vi "PathPlanner_Trajectory_GenerateStates_Pass3.vi"(9 "StartingSpeeds":T1 {"vOmega" format="%10.3f"; "vY" format="%10.3f"; "vX" format="%10.3f"}, 11 "in PathPlannerStates":T2[](array[typedef]) {"TargetHolonomicRotation"."SIN" format="%13.4f"; "TargetHolonomicRotation"."COS" format="%13.4f"; "TargetHolonomicRotation"."VALUE" format="%13.4f"; "Heading"."SIN" format="%13.4f"; "Heading"."COS" format="%13.4f"; "Heading"."VALUE" format="%13.4f"; "PositionMeters"."Y" format="%14.3f"; "PositionMeters"."X" format="%14.3f"}) -> (3 "out PathPlannerStates":T2[](array[typedef]) {"TargetHolonomicRotation"."SIN" format="%13.4f"; "TargetHolonomicRotation"."COS" format="%13.4f"; "TargetHolonomicRotation"."VALUE" format="%13.4f"; "Heading"."SIN" format="%13.4f"; "Heading"."COS" format="%13.4f"; "Heading"."VALUE" format="%13.4f"; "PositionMeters"."Y" format="%14.3f"; "PositionMeters"."X" format="%14.3f"})   [LabVIEW 2019, in "PathPlanner.lvlib"]
uses:
  PathPlanner.lvlib
  TypeDef/PathPlannerTrajectoryState.ctl
  <vilib>/Rock Robotics/WPI/ThirdParty/JAS_Junk/TrajLib/TypeDef/TRANSLATION2D.ctl
  <vilib>/Rock Robotics/WPI/ThirdParty/JAS_Junk/TrajLib/TypeDef/ROTATION2D.ctl
  TypeDef/PathPlannerPathConstraints.ctl
  <vilib>/Rock Robotics/WPI/ThirdParty/JAS_Junk/TrajLib/TypeDef/CHASSIS_SPEEDS.ctl
  <vilib>/Rock Robotics/WPI/ThirdParty/JAS_Junk/TrajLib/Rotation2d_UnaryMinus.vi
  <vilib>/Rock Robotics/WPI/ThirdParty/JAS_Junk/TrajLib/Rotation2d_RotateBy.vi
  <vilib>/Rock Robotics/WPI/ThirdParty/JAS_Junk/TrajLib/Rotation2d_CreateAngle.vi
  <vilib>/Rock Robotics/WPI/ThirdParty/JAS_Junk/TrajLib/Rotation2d_CreateXY.vi
  <vilib>/Rock Robotics/WPI/ThirdParty/JAS_Junk/TrajLib/Util_CalcDist.vi
  <vilib>/Rock Robotics/WPI/ThirdParty/JAS_Junk/TrajLib/Trajectory_Library.lvlib
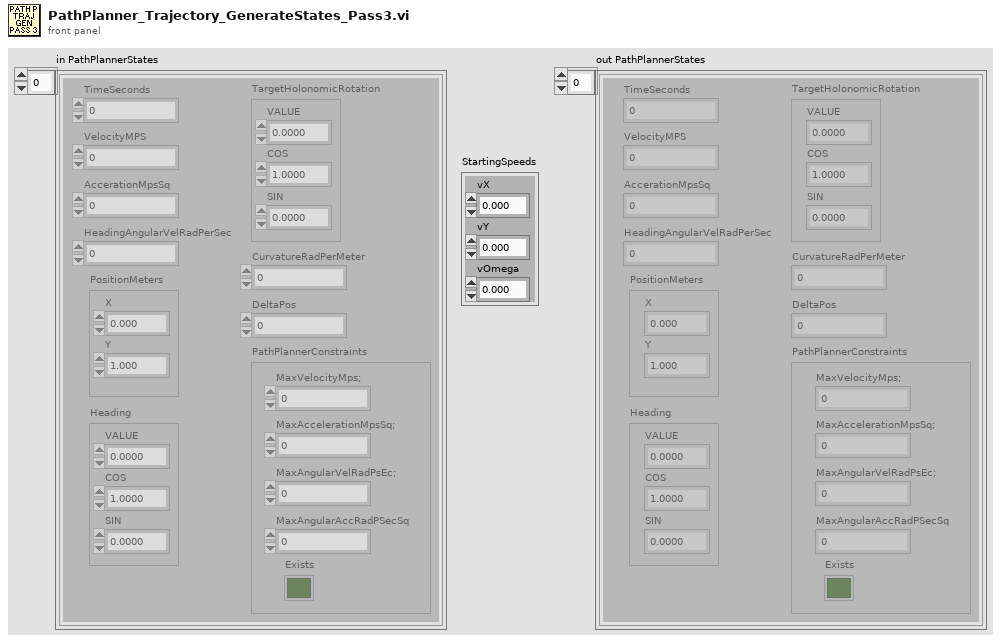
[diagram p1: front panel]
types:
  T1 = typedef "Trajectory_Library.lvlib/CHASSIS_SPEEDS.ctl" = cluster{"vX":dbl, "vY":dbl, "vOmega":dbl}
  T2 = typedef "PathPlanner.lvlib/PathPlannerTrajectoryState.ctl" = cluster{"TimeSeconds":dbl, "VelocityMPS":dbl, "AccerationMpsSq":dbl, "HeadingAngularVelRadPerSec":dbl, "PositionMeters":T3, "Heading":T4, "TargetHolonomicRotation":T4, "CurvatureRadPerMeter":dbl, "PathPlannerConstraints":T5, "DeltaPos":dbl}
  T3 = typedef "Trajectory_Library.lvlib/TRANSLATION2D.ctl" = cluster{"X":dbl, "Y":dbl}
  T4 = typedef "Trajectory_Library.lvlib/ROTATION2D.ctl" = cluster{"VALUE":dbl, "COS":dbl, "SIN":dbl}
  T5 = typedef "PathPlanner.lvlib/PathPlannerPathConstraints.ctl" = cluster{"MaxVelocityMps;":dbl, "MaxAccelerationMpsSq;":dbl, "MaxAngularVelRadPsEc;":dbl, "MaxAngularAccRadPSecSq":dbl, "Exists":bool}
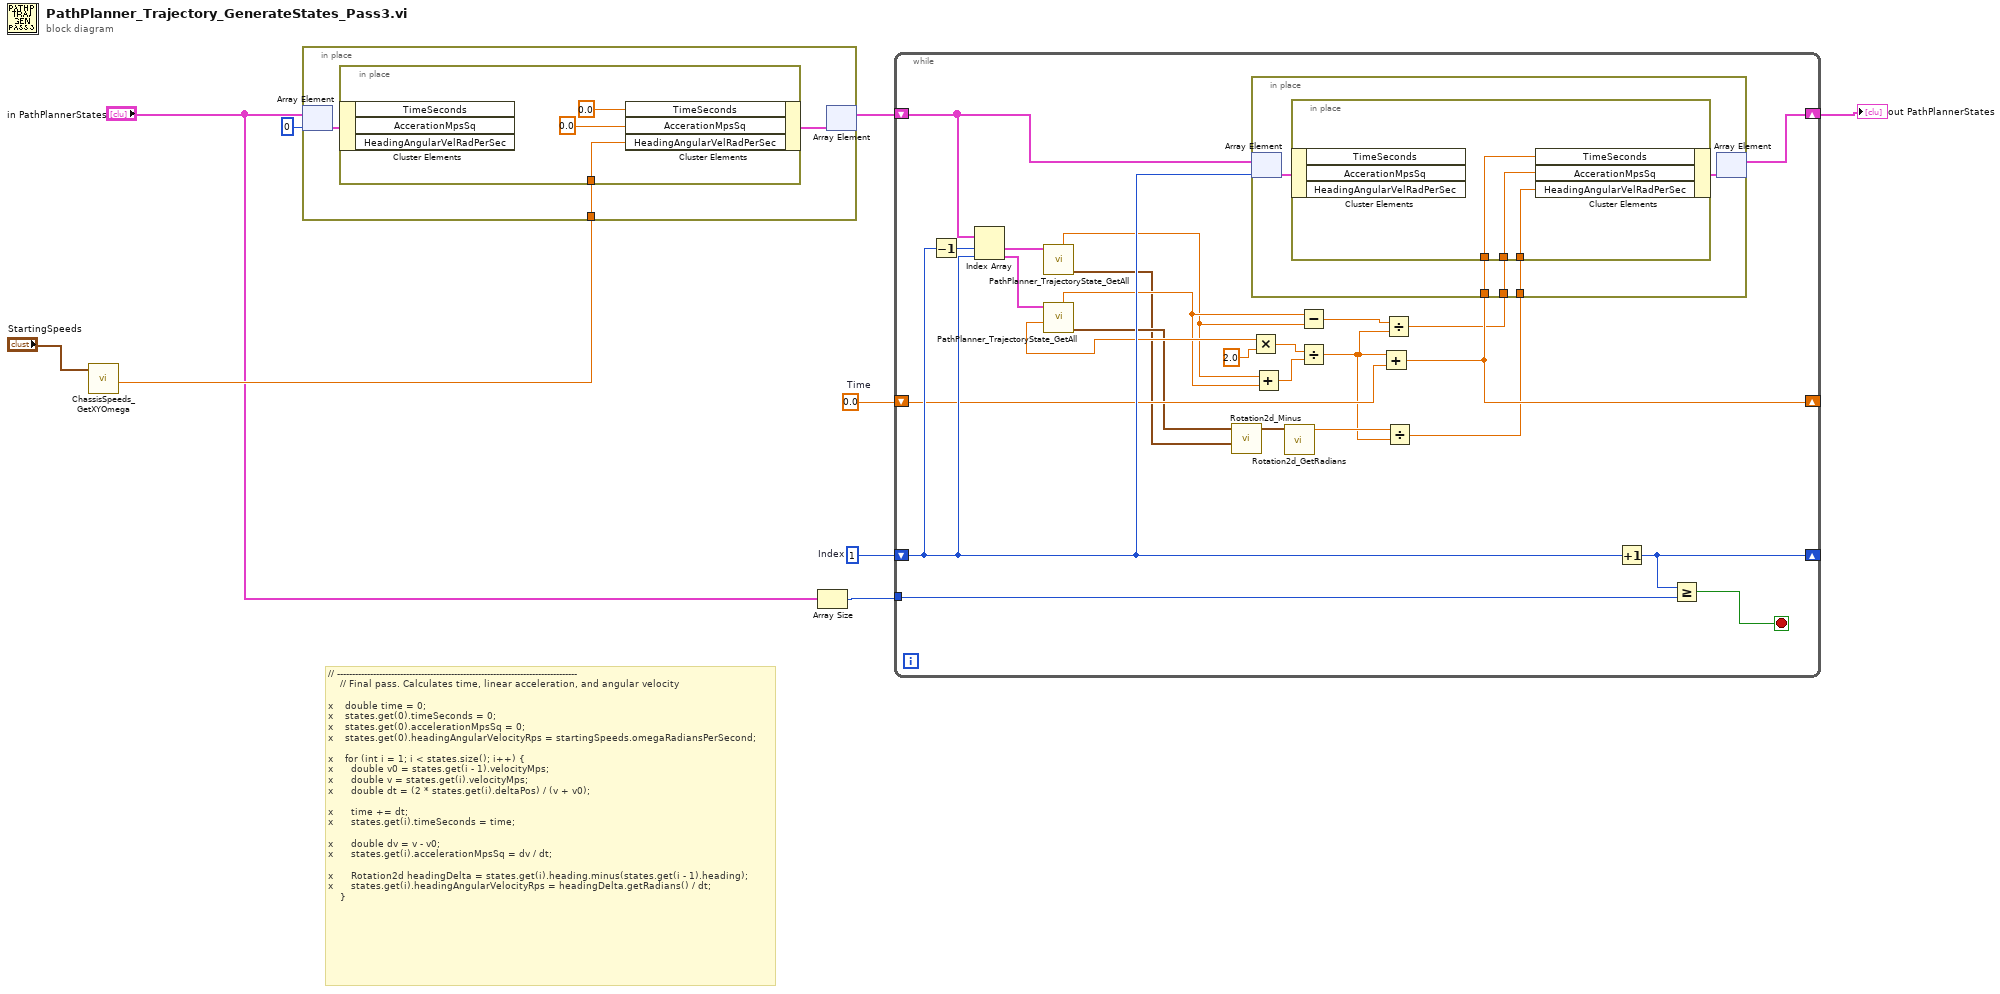
[diagram p0: block diagram]
diagram:
  w5 = 1  # Index
  w2 = 0.0  # Time
  # "// --------------------------------------------------------------------------------\n    // Final pass. Calculates time, linear acceleration, and angular velocity\n\nx    double time = 0;\nx    states.get(0).timeSeconds = 0;\nx    states.get(0).accelerationMpsSq = 0;\nx    states.get(0).headingAngularVelocityRps = startingSpeeds.omegaRadiansPerSecond;\n\nx    for (int i = 1; i < states.size(); i++) {\nx      double v0 = states.get(i - 1).velocityMps;\nx      double v = states.get(i).velocityMps;\nx      double dt = (2 * states.get(i).deltaPos) / (v + v0);\n\nx      time += dt;\nx      states.get(i).timeSeconds = time;\n\nx      double dv = v - v0;\nx      states.get(i).accelerationMpsSq = dv / dt;\n\nx      Rotation2d headingDelta = states.get(i).heading.minus(states.get(i - 1).heading);\nx      states.get(i).headingAngularVelocityRps = headingDelta.getRadians() / dt;\n    }"
  n1 = call <vilib>:"ChassisSpeeds_GetXYOmega.vi"("CHASSIS"="StartingSpeeds") -> ("vAngular"=w7:dbl)  [unwired: 8 in, 2 out]
  n2 = in-place {
    in-place-border: w7 -> [w10]
    n3 = in-place-array #1("in PathPlannerStates", 0) -> (w12:T2)
    n4 = in-place {
      in-place-border: w10 -> [w13]
      n5 = in-place-cluster #2(w12) -> ()  [unwired: 3 out]
      n6 = in-place-cluster #2("TimeSeconds"=0.0, "AccerationMpsSq"=0.0, "HeadingAngularVelRadPerSec"=w13) -> (w11:T2)
    }
    n7 = in-place-array #1(w11) -> (w6:T2[])  [unwired: 1 out]
  }
  n8 = Array Size(array="in PathPlannerStates") -> (size(s)=w3:i32)
  n9 = while {
    shift-right: [w37] -> w1
    shift-left: w6 -> [w35]
    shift-right: [w40] -> _
    shift-left: w5 -> [w32]
    tunnel: w3 -> [w39]
    shift-right: [w26] -> _
    shift-left: w2 -> [w27]
    stop <- w38 stop-if-true
    n10 = Decrement(x=w32) -> (x-1=w36:i32)
    n11 = Index Array(array=w35, index #1=w36, index #2=w32) -> (element #1=w34:T2, element #2=w33:T2)
    n12 = call "PathPlanner_TrajectoryState_GetAll.vi"("PathPlannerState"=w34) -> ("Heading"=w20:T4, "VelocityMPS"=w24:dbl)  [unwired: 1 in, 8 out]
    n13 = call "PathPlanner_TrajectoryState_GetAll.vi"("PathPlannerState"=w33) -> ("Heading"=w21:T4, "VelocityMPS"=w25:dbl, "DeltaPos"=w30:dbl)  [unwired: 1 in, 7 out]
    n14 = call <vilib>:"Rotation2d_Minus.vi"("other ROTATION"=w20, "in ROTATION"=w21) -> ("out ROTATION"=w19:T4)  [unwired: 9 in]
    n15 = Multiply(x=w30, y=2.0) -> (x*y=w29:dbl)
    n16 = Add(x=w24, y=w25) -> (x+y=w28:dbl)
    n17 = call <vilib>:"Rotation2d_GetRadians.vi"("in ROTATION"=w19) -> ("AngleRadians"=w18:dbl)  [unwired: 10 in]
    n18 = Subtract(x=w25, y=w24) -> (x-y=w23:dbl)
    n19 = Divide(x=w29, y=w28) -> (x/y=w17:dbl)
    n20 = Add(x=w17, y=w27) -> (x+y=w26:dbl)
    n21 = Divide(x=w23, y=w17) -> (x/y=w22:dbl)
    n22 = Divide(x=w18, y=w17) -> (x/y=w16:dbl)
    n23 = in-place {
      in-place-border: w26 -> [w43]
      in-place-border: w22 -> [w42]
      in-place-border: w16 -> [w41]
      n24 = in-place-array #3(w35, w32) -> (w45:T2)
      n25 = in-place {
        in-place-border: w43 -> [w48]
        in-place-border: w42 -> [w47]
        in-place-border: w41 -> [w46]
        n26 = in-place-cluster #4(w45) -> ()  [unwired: 3 out]
        n27 = in-place-cluster #4("TimeSeconds"=w48, "AccerationMpsSq"=w47, "HeadingAngularVelRadPerSec"=w46) -> (w44:T2)
      }
      n28 = in-place-array #3(w44) -> (w37:T2[])  [unwired: 1 out]
    }
    n29 = Increment(x=w32) -> (x+1=w40:i32)
    n30 = Greater Or Equal?(x=w40, y=w39) -> (x >= y?=w38:bool)
  }
  "out PathPlannerStates" <- w1
